vi "save_j-t_data.vi"(0 "Experiment Indicator":string, 1 "Cell details cluster":T1={"Cell Position"=16, "Cell Label"="", "Pixel to measure"=0, "Area (cm^2)"=0.126, "Variable"="", "Variable value"="", "Scan settings in queue"=0, "Light or dark"="", "Measurement Type"=""} {"Pixel to measure" items=["All", "1", "2", "3", "4", "5", "6", "7", "8"]}, 3 "Scan direction":i32, 4 "Data Array":dbl[][](array[numeric]), 6 "Username":string, 7 "Intensity (no. of suns)":string, 8 "Date array":string[](array[string])) -> (17 "File path for JV data":path, 18 "File path for JV image":path)   [LabVIEW 2016]
uses:
  <vilib>/Utility/file.llb/Write Delimited Spreadsheet (string).vi
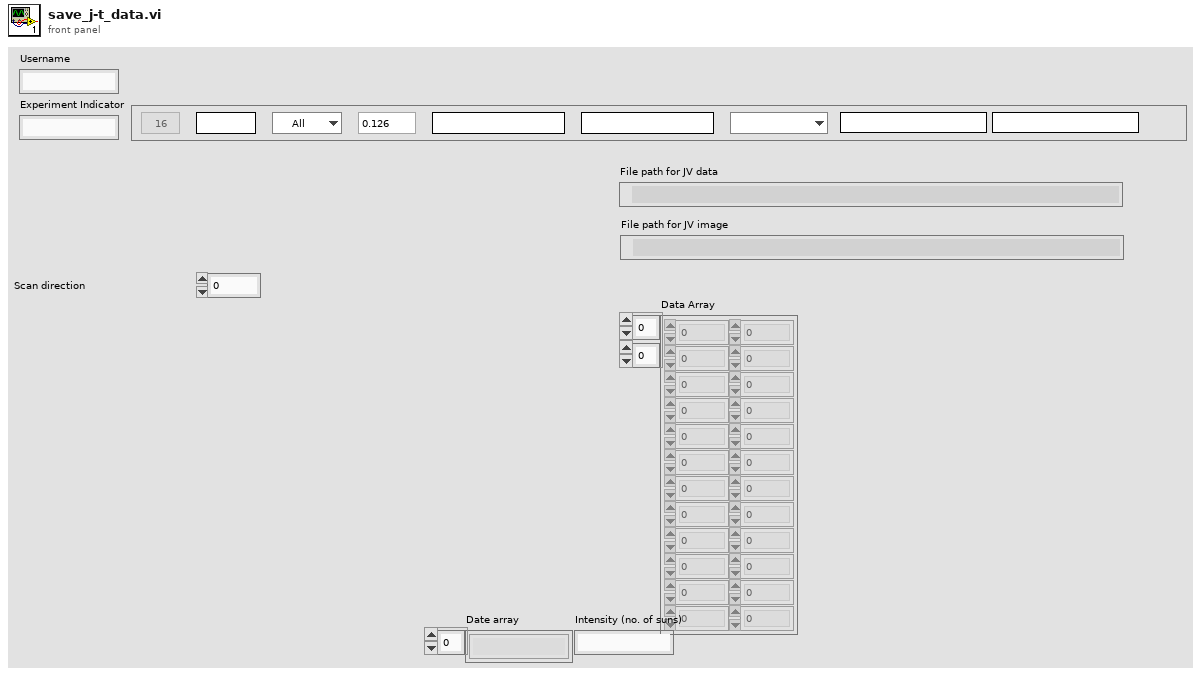
[diagram p1: front panel]
types:
  T1 = cluster{"Cell Position":i32, "Cell Label":string, "Pixel to measure":u16, "Area (cm^2)":dbl, "Variable":string, "Variable value":string, "Scan settings in queue":u16, "Light or dark":string, "Measurement Type":string}
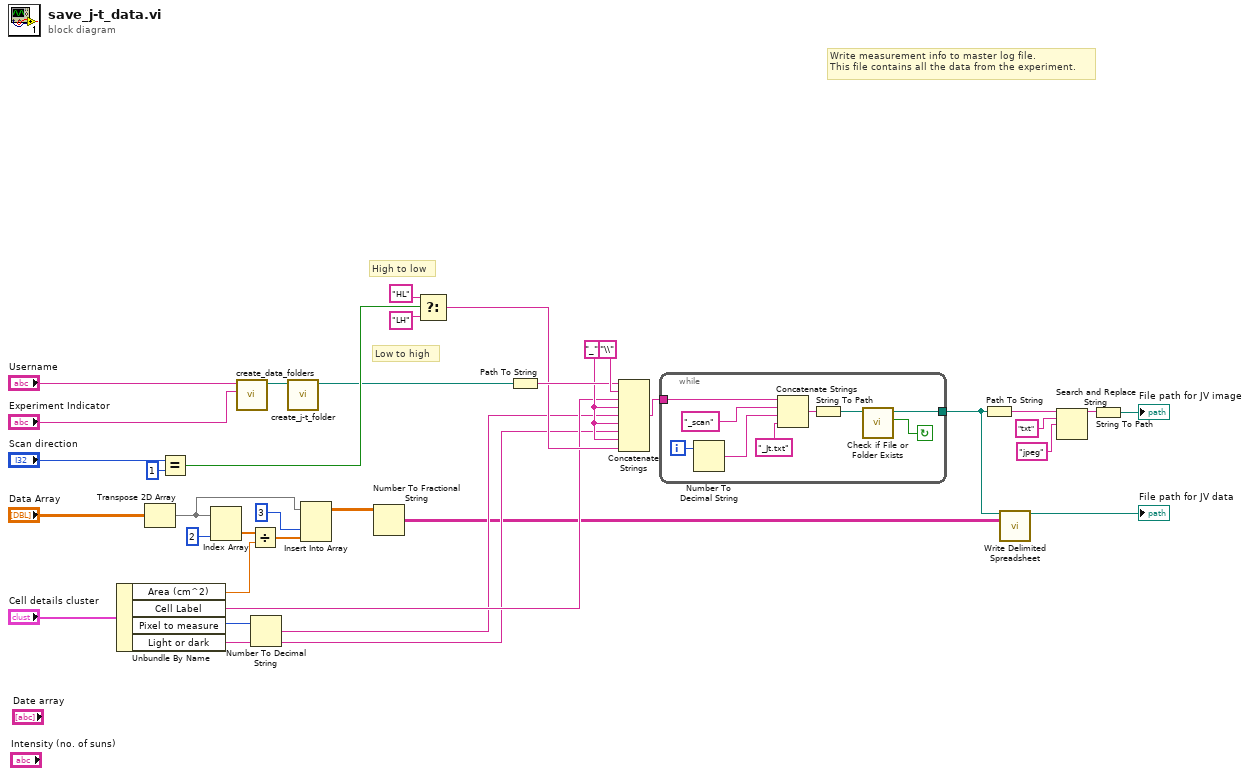
[diagram p0: block diagram]
diagram:
  w18 = "_"
  # "Write measurement info to master log file.\nThis file contains all the data from the experiment."
  # "Low to high"
  # "High to low"
  n1 = Unbundle By Name("Cell details cluster") -> ("Area (cm^2)"=w7:dbl, "Cell Label"=w6:string, "Pixel to measure"=w4:u16, "Light or dark"=w5:string)
  n2 = Transpose 2D Array(2D array="Data Array") -> (transposed array=w12:dbl[][])
  n3 = Equal?(x="Scan direction", y=1) -> (x = y?=w23:bool)
  n4 = Index Array(array=w12, index (col)=2) -> (element=w14:dbl[])  [unwired: 1 in]
  n5 = call "create_data_folders.vi"("Experiment Indicator"="Experiment Indicator", "username"="Username") -> ("Data Output Folder"=w9:path)  [unwired: 9 in]
  n6 = Divide(x=w14, y=w7) -> (x/y=w13:dbl[])
  n7 = Number To Decimal String(number=w4) -> (decimal integer string=w3:string)  [unwired: 1 in]
  n8 = call "create_j-t_folder.vi"("Data Folder In"=w9) -> ("Data Output Folder"=w8:path)  [unwired: 10 in]
  n9 = Insert Into Array(array=w12, index (col)=3, new element=w13) -> (w10:dbl[][])  [unwired: 1 in]
  n10 = Number To Fractional String(number=w10) -> (F-format string=w1:string[][])  [unwired: 3 in]
  n11 = Select(t="HL", s=w23, f="LH") -> (s? t:f=w17:string)
  n12 = Path To String(path=w8) -> (string=w32:string)
  n13 = Concatenate Strings(w32, "\\", w6, w18, w3, w18, w5, w18, w17) -> (w20:string)
  n14 = while {
    tunnel: w20 -> [w44]
    tunnel: [w36] -> w16
    i -> [w42]
    stop <- w37 continue-if-true
    n15 = Number To Decimal String(number=w42) -> (decimal integer string=w41:string)  [unwired: 1 in]
    n16 = Concatenate Strings(w44, "_scan", w41, "_Jt.txt") -> (w38:string)
    n17 = String To Path(string=w38) -> (path=w39:path)
    n18 = call <vilib>:"Check if File or Folder Exists.vi"("path"=w39) -> ("file or folder exists?"=w37:bool, "dup path"=w36:path)  [unwired: 8 in, 1 out]
  }
  n19 = Path To String(path=w16) -> (string=w19:string)
  n20 = call-poly <vilib>:"Write Delimited Spreadsheet.vi"("file path (dialog if empty)"=w16, "2D data"=w1) -> ("new file path (Not A Path if cancelled)"=→"File path for JV data":path)  [unwired: 12 in, 1 out]
  n21 = Search and Replace String(input string=w19, search string="txt", replace string="jpeg") -> (result string=w31:string)  [unwired: 5 in, 3 out]
  n22 = String To Path(string=w31) -> (path=→"File path for JV image":path)
